vi "Tracking Test DAA.vi"(8 "error in (no error)":errorcluster, 10 "Model in":refnum<class "Model.lvclass">, 11 "Test Actuator State in":refnum<class "Test Actuator State.lvclass">) -> (0 "error out":errorcluster, 1 "Pass":bool, 2 "Model out":refnum<class "Model.lvclass">, 3 "Test Actuator State out":refnum<class "Test Actuator State.lvclass">)   [LabVIEW 2016, in "Test Actuator State.lvclass"]
uses:
  Test Actuator State.lvclass
  Model/Model/Model.lvclass
  <vilib>/Platform/TimedLoop/XDataNode/timing_clust.ctl
  <vilib>/Platform/TimedLoop/XDataNode/nitl_modes.ctl
  <vilib>/Platform/TimedLoop/XDataNode/wakeup.ctl
  Model/Model/Model.lvclass/Model.ctl
  Typedefs/ActuatorSetPoints.ctl
  <vilib>/Analysis/5stat.llb/RMS (DBL).vi
  <vilib>/platform/TimedLoop/XDataNode/XDataNode.xnode
  Model/Waveforms/Waveform/Waveform.lvclass
  Typedefs/FAMT Typedefs.lvlib
  <vilib>/Analysis/NI_AALPro.lvlib
  <vilib>/Platform/TimedLoop/XDataNode/XDNodeRunTimeDep.lvlib
  <vilib>/Analysis/NI_AALBase.lvlib
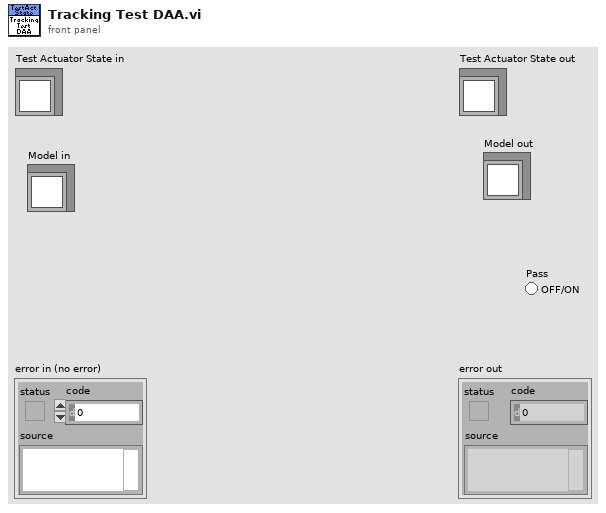
[diagram p1: front panel]
types:
  T1 = typedef "FAMT Typedefs.lvlib/TrackingTestSettings.ctl" = cluster{"Repeating Error (N)":dbl, "Process Time (s)":dbl, "Sample Time (s)":dbl, "Iterations":i32, "Amplitude (N)":dbl, "Non-Repeating Error":dbl}
  T2 = typedef "XDNodeRunTimeDep.lvlib/timing_clust.ctl" = cluster{"Expected End [f-1]":u64, "Actual End [f-1]":u64, "Finished Late? [f-1]":bool, "Expected End [i-1]":u64, "Actual End [i-1]":u64, "Finished Late? [i-1]":bool, "Expected Start [i]":u64, "Actual Start [i]":u64, "Expected Start [f]":u64, "Actual Start [f]":u64, "Source Name":string, "Structure Name":string, "Period":i64, "Deadline":i64, "Offset":i64, "Start":i64, "Priority":i32, "Timeout":i32, "Mode":T3, "Wakeup Reason":T4, "Error":errorcluster, "Source Type":string, "Secondary Source Type":string, "Global End Time":u64, "Global Start Time":u64, "Frame Duration":u64, "Iteration Duration":u64, "Assigned CPU":i32, "I/O Scan Engine Mode":u32}
  T3 = typedef "XDNodeRunTimeDep.lvlib/nitl_modes.ctl" = enum32{"No Change", "Process missed periods, maintain original phase", "Discard missed periods, maintain original phase", "Process missed periods, ignore original phase", "Discard missed periods, ignore original phase"}
  T4 = typedef "XDNodeRunTimeDep.lvlib/wakeup.ctl" = enum32{"Normal", "Aborted", "Asynchronous wakeup", "Timing source error", "Timed loop error", "Timeout"}
  T5 = typedef "FAMT Typedefs.lvlib/ActuatorSetPoints.ctl" = cluster{"Axial Force":dbl, "Lateral Force":dbl, "FC1 Force":dbl, "FC2 Force":dbl}
  T6 = typedef "FAMT Typedefs.lvlib/ActuatorData.ctl" = cluster{"Timestamp":dbl, "Axial Force":dbl, "Lateral Force":dbl, "FC1 Force":dbl, "FC2 Force":dbl, "Lateral Push Pressure":dbl, "Lateral Pull Pressure":dbl, "Axial Push Pressure":dbl, "Axial Pull Pressure":dbl}
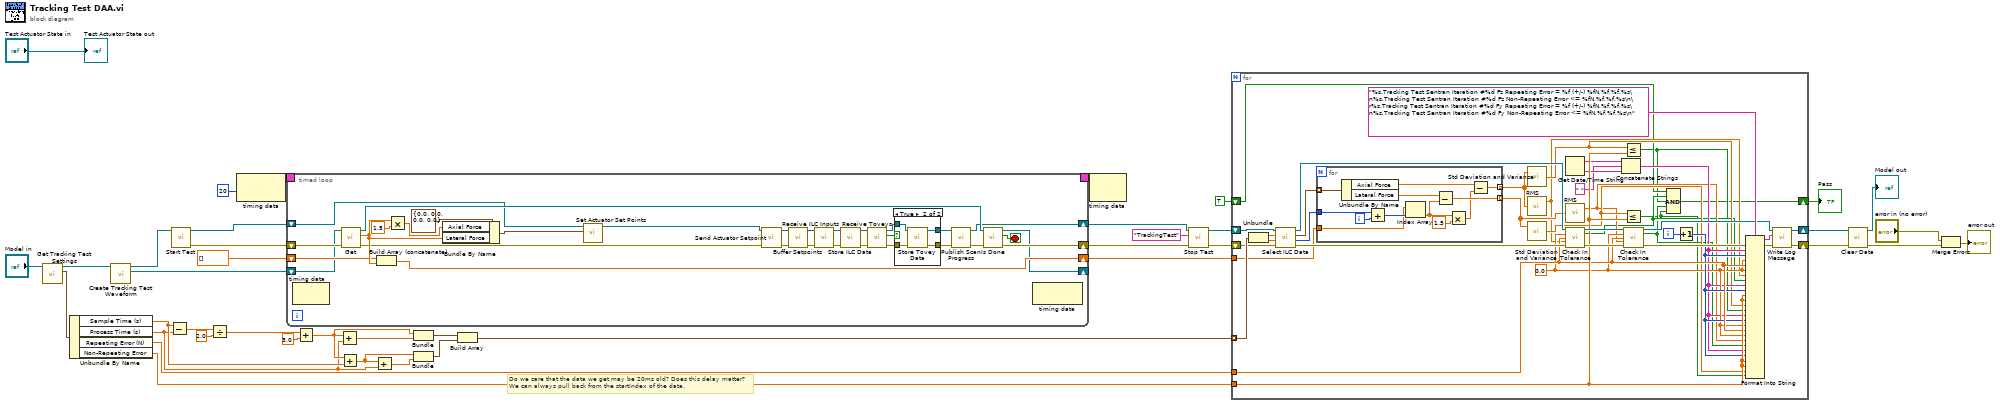
[diagram p0: block diagram]
diagram:
  # "Do we care that the data we get may be 20ms old? Does this delay matter?\nWe can always pull back from the startIndex of the data."
  n1 = call "Get Tracking Test Settings.vi"("Model in"="Model in") -> ("Tracking Test Settings"=w36:T1, "Model out"=w37:refnum<class "Model.lvclass">)  [unwired: 9 in]
  n2 = Unbundle By Name(w36) -> ("Sample Time (s)"=w24:dbl, "Process Time (s)"=w22:dbl, "Repeating Error (N)"=w33:dbl, "Non-Repeating Error"=w17:dbl)
  n3 = call "Create Tracking Test Waveform.vi"("Model in"=w37) -> ("Waveform"=w4:refnum<class "Waveform.lvclass">, "Model out"=w15:refnum<class "Model.lvclass">)  [unwired: 9 in]
  n4 = Subtract(x=w24, y=w22) -> (x-y=w30:dbl)
  n5 = call "Start Test.vi"("Model in"=w15) -> ("error out"=w6:errorcluster, "Model out"=w7:refnum<class "Model.lvclass">)  [unwired: 9 in]
  n6 = Divide(x=w30, y=2.0) -> (x/y=w28:dbl)
  n7 = node-c288(i64 20 ("Period")) -> (w10:T2)
  n8 = timed-loop {
    timing: w10 -> [_]
    timing-out: [_] -> w9
    shift-right: [w46] -> w3
    shift-left: w7 -> [w50]
    shift-right: [w45] -> w2
    shift-left: w6 -> [w49]
    shift-right: [w44] -> w1
    shift-left: dbl[] [] -> [w48]
    shift-right: [w43] -> _
    shift-left: w4 -> [w47]
    stop <- w42 stop-if-true
    n9 = node-c288() -> ()  [unwired: 1 in, 1 out]
    n10 = call-dynamic "Get.vi"("error in (no error)"=w49, "Waveform in"=w47) -> ("error out"=w64:errorcluster, "Value"=w70:dbl, "Waveform out"=w63:refnum<class "Waveform.lvclass">)  [unwired: 7 in]
    n11 = Build Array (concatenate)(w48, w70) -> (w44:dbl[])
    n12 = Multiply(x=w70, y=1.5) -> (x*y=w72:dbl)
    n13 = Bundle By Name(cluster=T5 {"Axial Force"=0.0, "Lateral Force"=0.0, "FC1 Force"=0.0, "FC2 Force"=0.0} ("Actuator Set Points"), "Axial Force"=w72, "Lateral Force"=w70) -> (w62:T5)
    n14 = call "Set Actuator Set Points.vi"("Actuator Set Points"=w62, "Model in"=w50) -> ("Model out"=w60:refnum<class "Model.lvclass">)  [unwired: 9 in]
    n15 = call "Send Actuator Setpoint.vi"("error in (no error)"=w64, "Model in"=w60) -> ("error out"=w69:errorcluster, "Model out"=w66:refnum<class "Model.lvclass">)  [unwired: 8 in]
    n16 = call "Buffer Setpoints.vi"("error in (no error)"=w69, "Model in"=w66) -> ("error out"=w68:errorcluster, "Model out"=w67:refnum<class "Model.lvclass">)  [unwired: 8 in]
    n17 = call "Receive ILC Inputs.vi"("error in (no error)"=w68, "Model in"=w67) -> ("error out"=w52:errorcluster, "Model out"=w51:refnum<class "Model.lvclass">)  [unwired: 8 in]
    n18 = call "Store ILC Data.vi"("error in (no error)"=w52, "Model in"=w51) -> ("error out"=w54:errorcluster, "Model out"=w53:refnum<class "Model.lvclass">)  [unwired: 8 in]
    n19 = call "Receive Toveys.vi"("error in (no error)"=w54, "Model in"=w53) -> ("error out"=w56:errorcluster, "Data Received"=w57:bool, "Model out"=w55:refnum<class "Model.lvclass">)  [unwired: 7 in]
    n20 = case shown="True" w57 {
      tunnel: w55 -> [w74 w78]
      tunnel: w56 -> [w73 w77]
      tunnel: [w73 w76] -> w59
      tunnel: [w74 w75] -> w58
      frame False {
      }
      frame True {
        n21 = call "Store Tovey Data.vi"("error in (no error)"=w77, "Model in"=w78) -> ("error out"=w76:errorcluster, "Model out"=w75:refnum<class "Model.lvclass">)  [unwired: 8 in]
      }
    }
    n22 = call "Publish Scan Progress.vi"("error in (no error)"=w59, "Model in"=w58) -> ("error out"=w65:errorcluster, "Model out"=w46:refnum<class "Model.lvclass">)  [unwired: 8 in]
    n23 = call-dynamic "Is Done.vi"("error in (no error)"=w65, "Waveform in"=w63) -> ("error out"=w45:errorcluster, "Is Done"=w42:bool, "Waveform out"=w43:refnum<class "Waveform.lvclass">)  [unwired: 7 in]
    n24 = node-c288() -> ()  [unwired: 1 in, 1 out]
  }
  n25 = Add(x=w28, y=3.0) -> (x+y=w25:dbl)
  n26 = Add(x=w25, y=w22) -> (x+y=w26:dbl)
  n27 = Add(x=w25, y=w24) -> (x+y=w23:dbl)
  n28 = Add(x=w23, y=w22) -> (x+y=w21:dbl)
  n29 = Bundle(w25, w26) -> (w20:cluster{dbl, dbl})  [unwired: 1 in]
  n30 = Bundle(w23, w21) -> (w19:cluster{dbl, dbl})  [unwired: 1 in]
  n31 = Build Array(w20, w19) -> (w18:cluster{dbl, dbl}[])
  n32 = node-c288(w9) -> ()  [unwired: 1 out]
  n33 = call "Stop Test.vi"("error in (no error)"=w2, "Test"="TrackingTest" ("format string"), "Model in"=w3) -> ("error out"=w13:errorcluster, "Model out"=w14:refnum<class "Model.lvclass">)  [unwired: 7 in]
  n34 = for {
    tunnel: w18 -> [w120] mode=indexing
    shift-right: [w108] -> w31
    shift-left: w14 -> [w119]
    shift-right: [w109] -> w32
    shift-left: w13 -> [w117]
    tunnel: w33 -> [w101]
    tunnel: w17 -> [w102]
    tunnel: w1 -> [w98]
    shift-right: [w81] -> w11
    shift-left: TRUE -> [w86]
    i -> [w111]
    w99 = 0.0
    n35 = Unbundle(w120) -> (w115:dbl, w114:dbl)
    n36 = call "Select ILC Data.vi"("error in (no error)"=w117, "End Time"=w114, "Start Time"=w115, "Model in"=w119) -> ("error out"=w113:errorcluster, "StartIndex"=w97:i32, "Data"=w118:T6[], "Model out"=w116:refnum<class "Model.lvclass">)  [unwired: 4 in]
    n37 = for {
      tunnel: w118 -> [w132] mode=indexing
      tunnel: [w130] -> w92 mode=indexing
      tunnel: [w128] -> w90 mode=indexing
      tunnel: w98 -> [w124]
      tunnel: w97 -> [w127]
      i -> [w126]
      n38 = Unbundle By Name(w132) -> ("Axial Force"=w131:dbl, "Lateral Force"=w129:dbl)
      n39 = Add(x=w127, y=w126) -> (x+y=w125:i32)
      n40 = Index Array(array=w124, index=w125) -> (element=w122:dbl)
      n41 = Subtract(x=w129, y=w122) -> (x-y=w128:dbl)
      n42 = Multiply(x=w122, y=1.5) -> (x*y=w121:dbl)
      n43 = Subtract(x=w131, y=w121) -> (x-y=w130:dbl)
    }
    n44 = call <vilib>:"Std Deviation and Variance.vi"("X"=w92) -> ("standard deviation"=w91:dbl)  [unwired: 1 in, 2 out]
    n45 = call-poly <vilib>:"RMS.vi"("X"=w92) -> ("rms value"=w88:dbl)  [unwired: 1 out]
    n46 = call <vilib>:"Std Deviation and Variance.vi"("X"=w90) -> ("standard deviation"=w89:dbl)  [unwired: 1 in, 2 out]
    n47 = Get Date/Time String() -> (date string=w95:string, time string=w94:string)  [unwired: 3 in]
    n48 = call-poly <vilib>:"RMS.vi"("X"=w90) -> ("rms value"=w87:dbl)  [unwired: 1 out]
    n49 = call "Check In Tolerance.vi"("Model in"=w116, "Expected"=w99, "Tolerance"=w101, "Actual"=w88, "error in (no error)"=w113) -> ("Model out"=w105:refnum<class "Model.lvclass">, "Pass"=w85:bool, "error out"=w106:errorcluster)  [unwired: 8 in]
    n50 = Concatenate Strings(w95, " " ("string"), w94) -> (w96:string)
    n51 = Less Or Equal?(x=w91, y=w102) -> (x <= y?=w84:bool)
    n52 = Less Or Equal?(x=w89, y=w102) -> (x <= y?=w82:bool)
    n53 = call "Check In Tolerance.vi"("Model in"=w105, "Expected"=w99, "Tolerance"=w101, "Actual"=w87, "error in (no error)"=w106) -> ("Model out"=w104:refnum<class "Model.lvclass">, "Pass"=w83:bool, "error out"=w103:errorcluster)  [unwired: 8 in]
    n54 = Compound Arithmetic op=AND(w86, w85, w84, w83, w82) -> (w81:bool)
    n55 = Increment(x=w111) -> (x+1=w100:i32)
    n56 = Format Into String(format string="%s,Tracking Test Sentran Iteration #%d Fz Repeating Error = %f (+/-) %fN,%f,%f,%s\n%s,Tracking Test Sentran Iteration #%d Fz Non-Repeating Error <= %fN,%f,%f,%s\n\r%s,Tracking Test Sentran Iteration #%d Fy Repeating Error = %f (+/-) %fN,%f,%f,%s\n%s,Tracking Test Sentran Iteration #%d Fy Non-Repeating Error <= %fN,%f,%f,%s\n", error in=w103, w96, w100, w99, w101, w99, w88, w85, w96, w100, w102, w102, w91, w84, w96, w100, w99, w101, w99, w87, w83, w96, w100, w102, w102, w89, w82) -> (resulting string=w107:string, error out=w110:errorcluster)  [unwired: 1 in]
    n57 = call "Write Log Message.vi"("error in (no error)"=w110, "Message"=w107, "Model in"=w104) -> ("error out"=w109:errorcluster, "Model out"=w108:refnum<class "Model.lvclass">)  [unwired: 7 in]
  }
  "Pass" <- w11
  n58 = call "Clear Data.vi"("error in (no error)"=w32, "Model in"=w31) -> ("error out"=w35:errorcluster, "Model out"=→"Model out":refnum<class "Model.lvclass">)  [unwired: 8 in]
  n59 = Merge Errors("error in (no error)", w35) -> (→"error out":errorcluster)
  "Test Actuator State out" <- "Test Actuator State in"
